vi "DestroySurface.vi"(8 "No Error":errorcluster, 11 "Surface [SDL_Surface *]":i64 format="%.0x") -> (0 "error out":errorcluster)   [LabVIEW 2026, in "SDL3.lvlib" / "Surface.lvlib"]
doc: "<B>Summary</B>\nFree a surface.\n\n<B>Remarks</B>\nIt is safe to pass NULL to this function."
uses:
  Surface.lvlib
  Lib/SDL3.dll
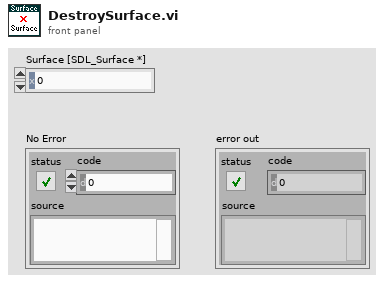
[diagram p1: front panel]
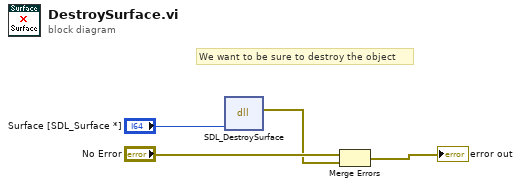
[diagram p0: block diagram]
diagram:
  # "We want to be sure to destroy the object"
  n1 = dll-call lib="C:/Users/saukko/Dev/LV-SDL3/Sources/SDL3/Lib/SDL3.*" fn="SDL_DestroySurface"("surface"="Surface [SDL_Surface *]") -> (error out=w1:errorcluster)  [unwired: 5 in, 1 out]
  n2 = Merge Errors("No Error", w1) -> (→"error out":errorcluster)
